vi "Maui.Config.GenerateFrameworkPath.vi"(8 "error in (no error)":errorcluster) -> (0 "error out":errorcluster, 3 "Framework Path":path, 4 "Path Created?":bool)   [LabVIEW 2019, in "Maui.Config.lvclass"]
uses:
  Maui.Config.lvclass
  <vilib>/Utility/sysdir.llb/System Directory Type.ctl
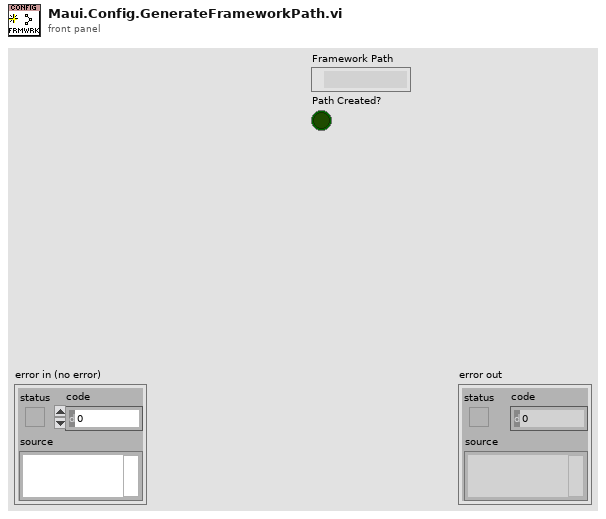
[diagram p1: front panel]
types:
  T1 = typedef "System Directory Type.ctl" = i32
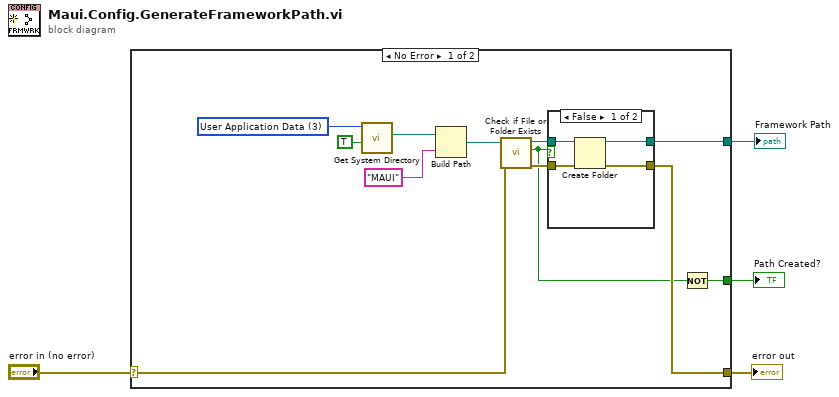
[diagram p0: block diagram]
diagram:
  n1 = case shown="No Error" "error in (no error)" {
    selector: "error in (no error)" -> [w9 w23]
    tunnel: [w8 w23] -> w3
    tunnel: [w7 _] -> w2
    tunnel: [w5 _] -> w1
    frame No Error {
      w16 = T1 3 items=["User Home"=0, "User Desktop"=1, "User Documents"=2, "User Application Data"=3, "User Preferences"=4, "User Temporary"=5, "Public Documents"=6, "Public Application Data"=7, "Public Preferences"=8, "Public Cache"=13, "System Core Libraries"=9, "System Installed Libraries"=10, "Application Files"=11, "Boot Volume Root"=12] ("system directory type")
      n2 = call <vilib>:"Get System Directory.vi"("create directory if not found? (F)"=TRUE, "system directory type"=w16) -> ("system directory"=w15:path)  [unwired: 9 in]
      n3 = Build Path(base path=w15, name or relative path="MAUI") -> (appended path=w12:path)
      n4 = call <vilib>:"Check if File or Folder Exists.vi"("error in (no error)"=w9, "path"=w12) -> ("error out"=w10:errorcluster, "file or folder exists?"=w6:bool, "dup path"=w11:path)  [unwired: 7 in]
      n5 = case shown="False" w6 {
        tunnel: w11 -> [w20 w22]
        tunnel: w10 -> [w19 w21]
        tunnel: [w18 w21] -> w8
        tunnel: [w17 w22] -> w7
        frame False {
          n6 = Create Folder(path (use dialog)=w20, error in=w19) -> (created path=w17:path, error out=w18:errorcluster)  [unwired: 1 in, 1 out]
        }
        frame True {
        }
      }
      n7 = Not(x=w6) -> (.not. x?=w5:bool)
    }
    frame Error {
    }
  }
  "error out" <- w3
  "Framework Path" <- w2
  "Path Created?" <- w1
